vi "Initialize Transfer Groups.vi"(5 "Transfer Group Status":refnum<class "Status.lvclass">, 7 "FIFO Options":T1, 8 "error in (no error)":errorcluster, 10 "Transfer Group configurations":T2[](array[typedef]) {"Transfers"."channels"."string offset" format="%d bytes"}, 11 "Plugin in":refnum<class "Plugin.lvclass">) -> (0 "error out":errorcluster, 2 "Transfer Groups":refnum<class "Transfer Group.lvclass">[](array[class]), 3 "Plugin out":refnum<class "Plugin.lvclass">)   [LabVIEW 2017, in "DSF Core.lvlib" / "Plugin.lvclass"]
uses:
  Plugin.lvclass
  Typedefs/DSF Engine Transfer Group Configuration.ctl
  Typedefs/DSF Direction.ctl
  Typedefs/DSF Timing Info.ctl
  Typedefs/DSF Settings Info.ctl
  Typedefs/DSF Engine Transfer Configuration.ctl
  Typedefs/DSF Byte Order.ctl
  Typedefs/DSF Engine Channel Configuration.ctl
  Typedefs/DSF Data Type.ctl
  Typedefs/DSF Timeout Behavior.ctl
  Transfer Group/Transfer Group.lvclass
  Typedefs/DSF FIFO Options.ctl
  Status/Status.lvclass
  Plugin.lvclass/Plugin.ctl
  Configuration/Required Buffer Size (Transfer Group).vi
  Configuration/Configuration Session.lvclass
  Buffers/Buffers.lvclass
  Timing/Timing.lvclass
  DSF Core.lvlib
  Framework/Framework.lvclass
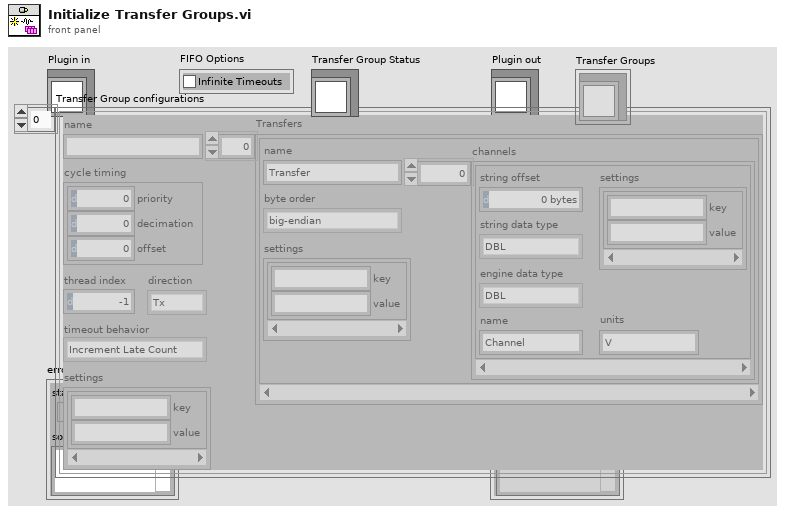
[diagram p1: front panel]
types:
  T1 = typedef "DSF Core.lvlib/Framework.lvclass/DSF FIFO Options.ctl" = cluster{"Infinite Timeouts":bool}
  T2 = typedef "DSF Core.lvlib/DSF Engine Transfer Group Configuration.ctl" = cluster{"name":string, "direction":T3, "cycle timing":T4, "thread index":i32, "settings":T5, "Transfers":T6[], "timeout behavior":T10}
  T3 = typedef "DSF Core.lvlib/DSF Direction.ctl" = enum8{"Tx", "Rx"}
  T4 = typedef "DSF Core.lvlib/DSF Timing Info.ctl" = cluster{"priority":u64, "decimation":u64, "offset":u64}
  T5 = typedef "DSF Core.lvlib/DSF Settings Info.ctl" = cluster{"key":string, "value":string}[]
  T6 = typedef "DSF Core.lvlib/DSF Engine Transfer Configuration.ctl" = cluster{"name":string, "byte order":T7, "settings":T5, "channels":T8[]}
  T7 = typedef "DSF Core.lvlib/DSF Byte Order.ctl" = enum8{"big-endian", "little-endian"}
  T8 = typedef "DSF Core.lvlib/DSF Engine Channel Configuration.ctl" = cluster{"string offset":u64, "string data type":T9, "engine data type":T9, "name":string, "settings":T5, "units":string}
  T9 = typedef "DSF Core.lvlib/DSF Data Type.ctl" = enum8{"Bool", "SGL", "DBL", "I8", "I16", "I32", "I64", "U8", "U16", "U32", "U64"}
  T10 = typedef "DSF Core.lvlib/DSF Timeout Behavior.ctl" = enum8{"Increment Late Count", "Throw Error"}
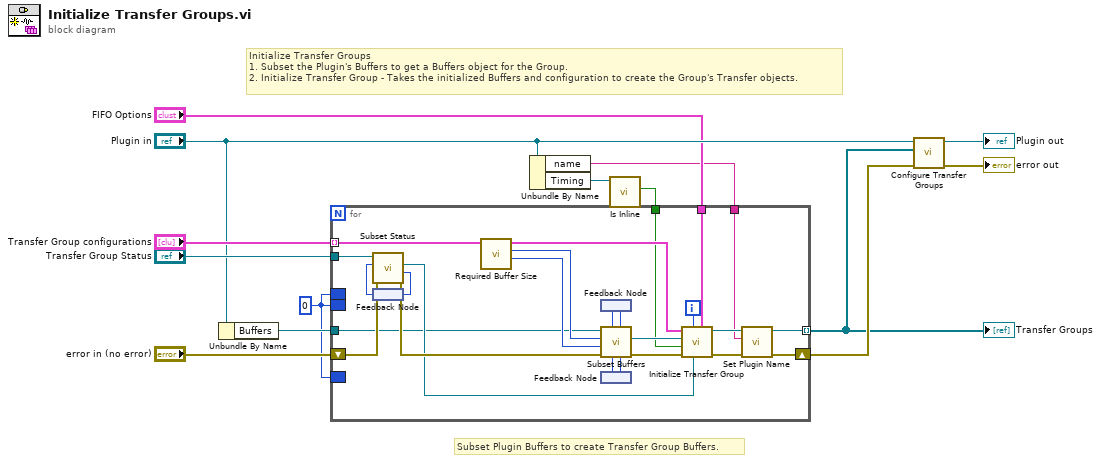
[diagram p0: block diagram]
diagram:
  w4 = u64 0 ("string buffer offset")
  # "Initialize Transfer Groups\n1. Subset the Plugin's Buffers to get a Buffers object for the Group.\n2. Initialize Transfer Group - Takes the initialized Buffers and configuration to create the Group's Transfer objects."
  # "Subset Plugin Buffers to create Transfer Group Buffers."
  n1 = Unbundle By Name("Plugin in") -> ("Buffers"=w6:refnum<class "Buffers.lvclass">)
  n2 = Unbundle By Name("Plugin in") -> ("name"=w1:string, "Timing"=w9:refnum<class "Timing.lvclass">)
  n3 = call "Is Inline.vi"("Timing in"=w9) -> ("inline?"=w11:bool)  [unwired: 9 in, 1 out]
  n4 = for {
    shift-right: [w38] -> w12
    shift-left: "error in (no error)" -> [w23]
    tunnel: [w26] -> w10 mode=indexing
    tunnel: w6 -> [w15]
    border: w4 -> [_]
    border: w4 -> [_]
    tunnel: "Transfer Group configurations" -> [w36] mode=indexing
    tunnel: w11 -> [w29]
    tunnel: "FIFO Options" -> [w28]
    tunnel: w1 -> [w25]
    tunnel: "Transfer Group Status" -> [w24]
    border: w4 -> [_]
    i -> [w19]
    n5 = feedback #1() -> (w17:u64)
    n6 = call "Subset Status.vi"("error in (no error)"=w23, "index"=w17, "status pointer in"=w24) -> ("error out"=w22:errorcluster, "index + count"=w18:u64, "subset status pointer"=w16:refnum<class "Status.lvclass">)  [unwired: 5 in, 1 out]
    n7 = feedback-in #1(w18) -> ()
    n8 = call-poly "Required Buffer Size.vi"("Transfer Group Configuration in"=w36) -> ("total engine buffer size"=w21:u64, "total string buffer size"=w20:u64, "Transfer Group Configuration out"=w37:T2)  [unwired: 7 in, 1 out]
    n9 = feedback #2() -> (w31:u64)
    n10 = feedback #3() -> (w33:u64)
    n11 = call "Subset Buffers.vi"("inline buffer offset"=w33, "string buffer offset"=w31, "error in (no error)"=w22, "inline buffer size"=w21, "string buffer size"=w20, "Buffers in"=w15) -> ("error out"=w35:errorcluster, "subset Buffers"=w30:refnum<class "Buffers.lvclass">, "inline buffer offset +size"=w34:u64, "string buffer offset + size"=w32:u64)  [unwired: 1 in, 1 out]
    n12 = feedback-in #2(w32) -> ()
    n13 = feedback-in #3(w34) -> ()
    n14 = call "Initialize Transfer Group.vi"("FIFO Options"=w28, "Transfer Group Status"=w16, "id"=w19, "error in (no error)"=w35, "force inline? (F)"=w29, "Transfer Group Buffers"=w30, "Transfer Group Configuration"=w37) -> ("error out"=w38:errorcluster, "Transfer Group out"=w27:refnum<class "Transfer Group.lvclass">)  [unwired: 3 in]
    n15 = call "Set Plugin Name.vi"("plugin"=w25, "Transfer Group in"=w27) -> ("Transfer Group out"=w26:refnum<class "Transfer Group.lvclass">)  [unwired: 9 in]
  }
  "Transfer Groups" <- w10
  n16 = call "Configure Transfer Groups.vi"("error in (no error)"=w12, "Transfer Groups"=w10, "Plugin in"="Plugin in") -> ("error out"=→"error out":errorcluster, "Plugin out"=→"Plugin out":refnum<class "Plugin.lvclass">)  [unwired: 7 in]
